vi "__init__.vi"(8 "error in":errorcluster, 9 "Function Generator":refnum<class "Function Generator.lvclass">, 10 "PZT":refnum<class "PZT.lvclass">, 11 "Lock-In Amplifier":refnum<class "Lock-In Amplifier.lvclass">) -> (0 "error out":errorcluster, 3 "Approach Curve out":refnum<class "Approach Curve.lvclass">)   [LabVIEW 2020, in "Approach Curve.lvclass"]
uses:
  Approach Curve.lvclass
  Lock-In Amplifier/Lock-In Amplifier.lvclass
  PZT/PZT.lvclass
  Function Generator/Function Generator.lvclass
panel:
  # "Need to \n1) Set function generator amplitude, frequency\n\n2) Calculate free amplitude\n\n3) Autophase?"
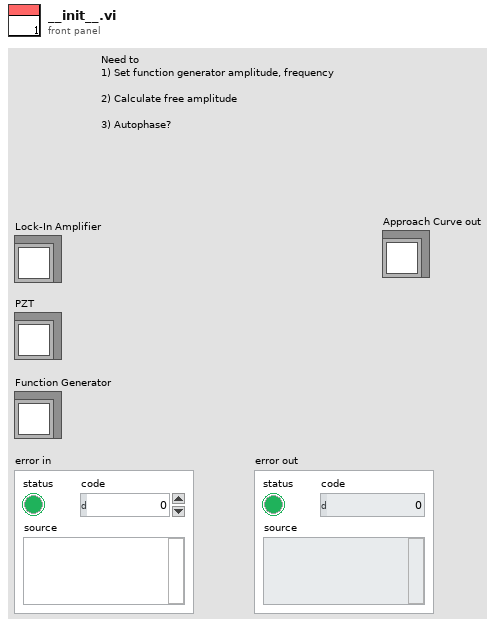
[diagram p1: front panel]
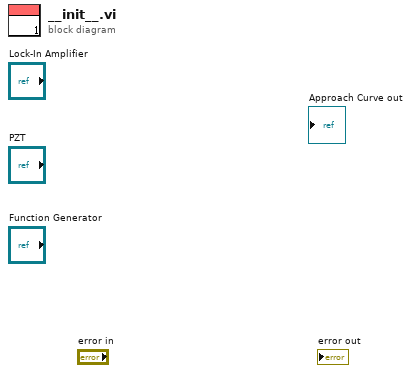
[diagram p0: block diagram]
diagram:
